vi "Ack_Nack Bit.vi"(8 "error in (no error)":errorcluster, 11 "Low Speed in":refnum<class "Low Speed.lvclass">) -> (0 "error out":errorcluster, 3 "Low Speed out":refnum<class "Low Speed.lvclass">)   [LabVIEW 2020, in "Low Speed.lvclass"]
uses:
  Low Speed.lvclass
  C:/Users/kaiser.asan/OneDrive - SolitonTechnologies/LabVIEW/29.SDLC - I2C Driver/I2C Module/I2C Controller Module/Class/Transmission Mode/Parent/TX Speed.lvclass
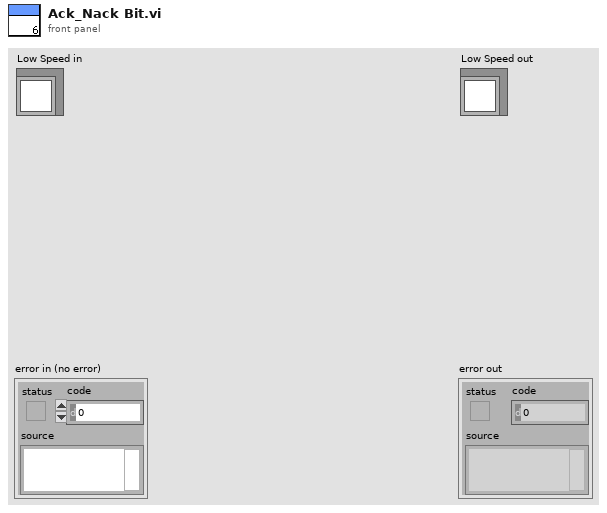
[diagram p1: front panel]
types:
  T1 = typedef "I2C Controller Lib.lvlib/Timing Parameters Cluster.ctl" = cluster{"f_SCL(KHz)":u32, "t_HIGH (ns)":u32, "t_LOW (ns)":u32, "t_SU;STA (ns)":u32, "t_HD;STA (ns)":u32, "t_SU;DAT (ns)":u32, "t_HD;DAT (ns)":u32, "t_SU;STO (ns)":u32, "t_BUF (ns)":u32}
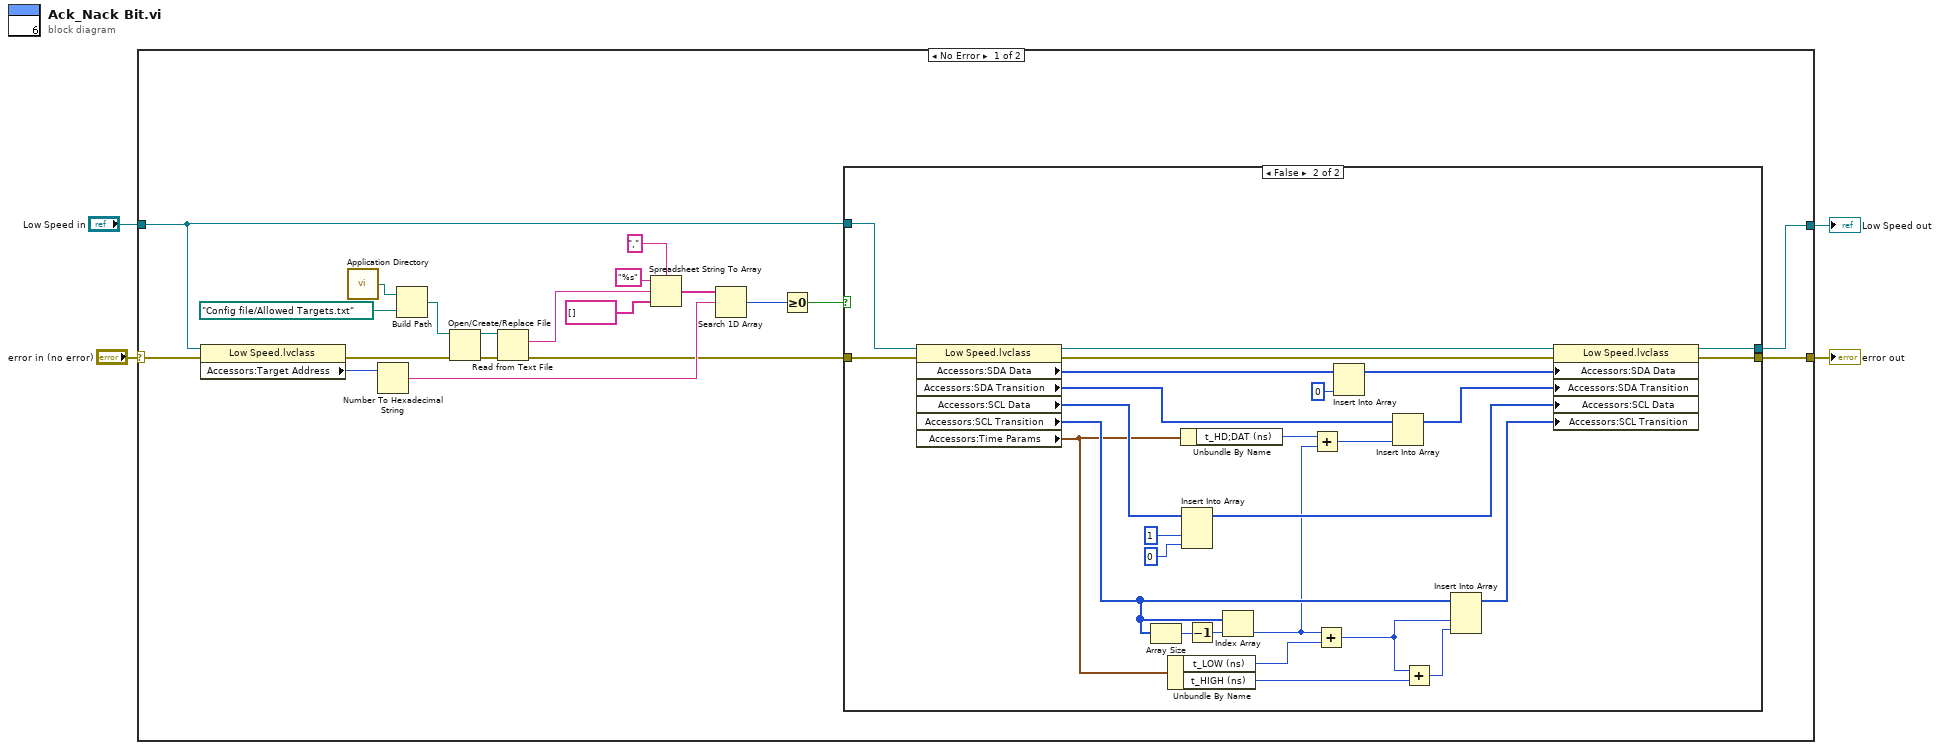
[diagram p0: block diagram]
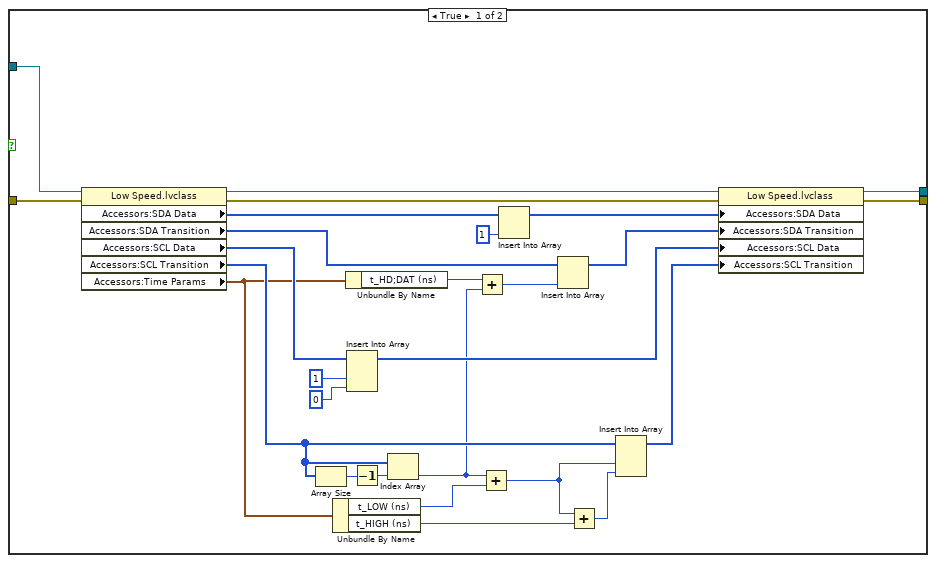
[diagram p2: hidden frame]
diagram:
  n1 = case shown="No Error" "error in (no error)" {
    selector: "error in (no error)" -> [w22 w80]
    tunnel: [w8 w80] -> w4
    tunnel: [w7 w79] -> w3
    tunnel: "Low Speed in" -> [w9 w79]
    frame No Error {
      n2 = property class="Low Speed.lvclass"(reference=w9, error in=w22) -> (error out=w21:errorcluster, "Accessors:Target Address"=w14:u16)  [unwired: 1 out]
      n3 = call <vilib>:"Application Directory.vi"() -> ("Application Directory"=w24:path)
      n4 = Number To Hexadecimal String(2:w14) -> (0:w13:string)  [unwired: 1 in]
      n5 = Build Path(base path=w24, name or relative path=path "Config file/Allowed Targets.txt" ("Application Directory")) -> (appended path=w20:path)
      n6 = Open/Create/Replace File(file path (use dialog)=w20, error in=w21) -> (refnum out=w18:refnum<file>, error out=w19:errorcluster)  [unwired: 4 in, 1 out]
      n7 = Read from Text File(file (use dialog)=w18, error in=w19) -> (text=w17:string, error out=w10:errorcluster)  [unwired: 2 in, 2 out]
      n8 = Spreadsheet String To Array(delimiter (Tab)=",", format string="%s", spreadsheet string=w17, array type (2D Dbl)=string[] [] ("text")) -> (array=w15:string[])
      n9 = Search 1D Array(1D array=w15, element=w13) -> (index of element=w12:i32)  [unwired: 1 in]
      n10 = Greater Or Equal To 0?(x=w12) -> (x >= 0?=w11:bool)
      n11 = case shown="False" w11 {
        tunnel: w10 -> [w28 w55]
        tunnel: w9 -> [w26 w53]
        tunnel: [w27 w54] -> w8
        tunnel: [w25 w52] -> w7
        frame True {
          n12 = property class="Low Speed.lvclass"(reference=w26, error in=w28) -> (reference out=w48:refnum<class "Low Speed.lvclass">, error out=w51:errorcluster, "Accessors:SDA Data"=w37:u8[], "Accessors:SDA Transition"=w32:u32[], "Accessors:SCL Data"=w47:u8[], "Accessors:SCL Transition"=w39:u32[], "Accessors:Time Params"=w33:T1)
          n13 = Array Size(array=w39) -> (size(s)=w45:i32)
          n14 = Unbundle By Name(w33) -> ("t_LOW (ns)"=w43:u32, "t_HIGH (ns)"=w42:u32)
          n15 = Unbundle By Name(w33) -> ("t_HD;DAT (ns)"=w30:u32)
          n16 = Insert Into Array(array=w47, new element #1=u8 1 ("new element/subarray"), new element #2=u8 0 ("new element/subarray")) -> (w46:u8[])  [unwired: 1 in]
          n17 = Decrement(x=w45) -> (x-1=w44:i32)
          n18 = Index Array(array=w39, index=w44) -> (element=w29:u32)
          n19 = Add(x=w30, y=w29) -> (x+y=w34:u32)
          n20 = Add(x=w29, y=w43) -> (x+y=w40:u32)
          n21 = Insert Into Array(array=w37, new element=u8 1 ("new element/subarray")) -> (w36:u8[])  [unwired: 1 in]
          n22 = Insert Into Array(array=w32, new element=w34) -> (w31:u32[])  [unwired: 1 in]
          n23 = Add(x=w40, y=w42) -> (x+y=w41:u32)
          n24 = Insert Into Array(array=w39, new element #1=w40, new element #2=w41) -> (w38:u32[])  [unwired: 1 in]
          n25 = property class="Low Speed.lvclass"(reference=w48, error in=w51, "Accessors:SDA Data"=w36, "Accessors:SDA Transition"=w31, "Accessors:SCL Data"=w46, "Accessors:SCL Transition"=w38) -> (reference out=w25:refnum<class "Low Speed.lvclass">, error out=w27:errorcluster)
        }
        frame False {
          n26 = property class="Low Speed.lvclass"(reference=w53, error in=w55) -> (reference out=w75:refnum<class "Low Speed.lvclass">, error out=w78:errorcluster, "Accessors:SDA Data"=w64:u8[], "Accessors:SDA Transition"=w59:u32[], "Accessors:SCL Data"=w74:u8[], "Accessors:SCL Transition"=w66:u32[], "Accessors:Time Params"=w60:T1)
          n27 = Array Size(array=w66) -> (size(s)=w72:i32)
          n28 = Unbundle By Name(w60) -> ("t_LOW (ns)"=w70:u32, "t_HIGH (ns)"=w69:u32)
          n29 = Unbundle By Name(w60) -> ("t_HD;DAT (ns)"=w57:u32)
          n30 = Insert Into Array(array=w74, new element #1=u8 1 ("new element/subarray"), new element #2=u8 0 ("new element/subarray")) -> (w73:u8[])  [unwired: 1 in]
          n31 = Decrement(x=w72) -> (x-1=w71:i32)
          n32 = Index Array(array=w66, index=w71) -> (element=w56:u32)
          n33 = Add(x=w57, y=w56) -> (x+y=w61:u32)
          n34 = Add(x=w56, y=w70) -> (x+y=w67:u32)
          n35 = Insert Into Array(array=w64, new element=u8 0 ("new element/subarray")) -> (w63:u8[])  [unwired: 1 in]
          n36 = Insert Into Array(array=w59, new element=w61) -> (w58:u32[])  [unwired: 1 in]
          n37 = Add(x=w67, y=w69) -> (x+y=w68:u32)
          n38 = Insert Into Array(array=w66, new element #1=w67, new element #2=w68) -> (w65:u32[])  [unwired: 1 in]
          n39 = property class="Low Speed.lvclass"(reference=w75, error in=w78, "Accessors:SDA Data"=w63, "Accessors:SDA Transition"=w58, "Accessors:SCL Data"=w73, "Accessors:SCL Transition"=w65) -> (reference out=w52:refnum<class "Low Speed.lvclass">, error out=w54:errorcluster)
        }
      }
    }
    frame Error {
    }
  }
  "error out" <- w4
  "Low Speed out" <- w3
